vi "String.Generate CRC.vi"(7 "Hex":bool, 10 "NumChars":i32=4, 11 "String":string) -> (2 "CRC String":string, 3 "CRC":i32)   [LabVIEW 2019]
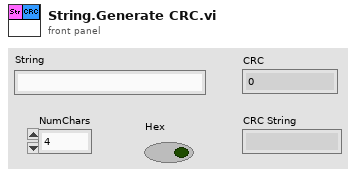
[diagram p1: front panel]
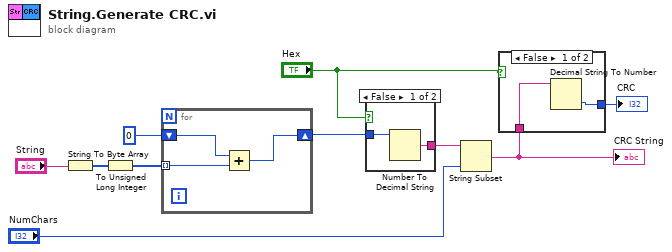
[diagram p0: block diagram]
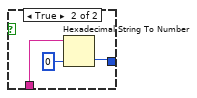
[diagram p2: hidden frame]
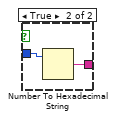
[diagram p3: hidden frame]
diagram:
  n1 = String To Byte Array(string="String") -> (unsigned byte array=w8:u8[])
  n2 = To Unsigned Long Integer(number=w8) -> (unsigned 32bit integer=w7:u32[])
  n3 = for {
    shift-right: [w11] -> w6
    shift-left: u32 0 -> [w13]
    tunnel: w7 -> [w12] mode=indexing
    n4 = Add(x=w13, y=w12) -> (x+y=w11:u32)
  }
  n5 = case shown="False" "Hex" {
    tunnel: w6 -> [w15 w17]
    tunnel: [w14 w16] -> w5
    frame False {
      n6 = Number To Decimal String(number=w15) -> (decimal integer string=w14:string)  [unwired: 1 in]
    }
    frame True {
      n7 = Number To Hexadecimal String(2:w17) -> (0:w16:string)  [unwired: 1 in]
    }
  }
  n8 = String Subset(string=w5, length (rest)="NumChars") -> (substring=w3:string)  [unwired: 1 in]
  "CRC String" <- w3
  n9 = case shown="False" "Hex" {
    tunnel: [w19 w22] -> w4
    tunnel: w3 -> [w18 w21]
    frame False {
      n10 = Decimal String To Number(string=w18) -> (number=w19:i32)  [unwired: 2 in, 1 out]
    }
    frame True {
      n11 = Hexadecimal String To Number(string=w21, default (0uL)=0 ("default (0 U32)")) -> (number=w22:i32)  [unwired: 1 in, 1 out]
    }
  }
  "CRC" <- w4
